vi "Fetch ALL.vi"(8 "error in":errorcluster, 11 "VISA resource name":refnum<visa-resource-name>) -> (0 "error out":errorcluster, 1 "Measurement":string, 3 "VISA resource name out":refnum<visa-resource-name>)   [LabVIEW 2020, in "IT-M7700.lvlib"]
doc: "The command is used to read in the memory Vrms, Vdc, Irms, Idc, Ipk_plus, Ipk_minus, W (Real Power), PF, IPmax, VA, Q (VAR), VTHD, Freq, Vpeak, VAC, IAC, ITHD17 set of values."
uses:
  <instrlib>/IT-M7700/IT-M7700.lvlib
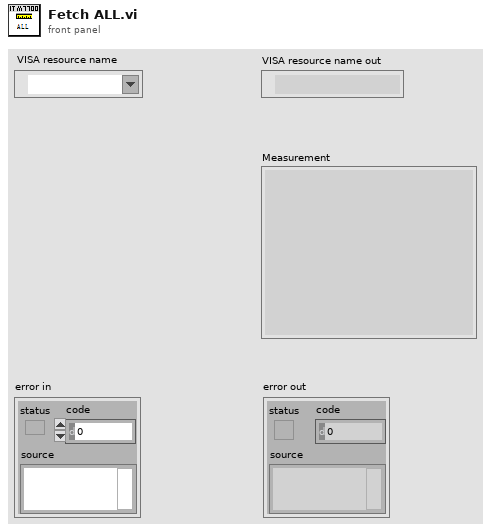
[diagram p1: front panel]
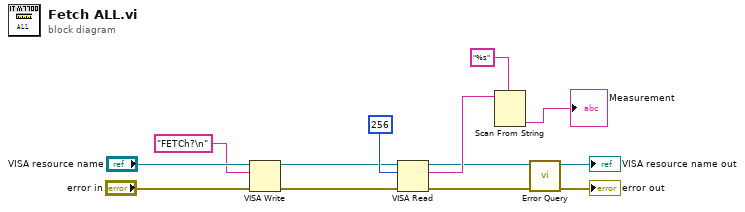
[diagram p0: block diagram]
diagram:
  n1 = VISA Write(VISA resource name="VISA resource name", write buffer="FETCh?\n", error in (no error)="error in") -> (VISA resource name out=w3:refnum<visa-resource-name>, error out=w2:errorcluster)  [unwired: 1 out]
  n2 = VISA Read(VISA resource name=w3, byte count=256, error in (no error)=w2) -> (VISA resource name out=w8:refnum<visa-resource-name>, read buffer=w13:string, error out=w4:errorcluster)  [unwired: 1 out]
  n3 = Scan From String(format string="%s", input string=w13) -> (output 1=→"Measurement":string)  [unwired: 3 in, 3 out]
  n4 = call <instrlib>:"Error Query.vi"("error in"=w4, "VISA resource name"=w8) -> ("error out"=→"error out":errorcluster, "VISA resource name out"=→"VISA resource name out":refnum<visa-resource-name>)  [unwired: 6 in, 2 out]
